vi "Read Write Exclude path.vi"(0 "path In":path, 5 "Key In":string, 7 "Exclude Path In":path[](array[path]), 11 "Error In":errorcluster, 13 "Write?":bool) -> (4 "Path Out":path, 6 "Key out":string, 8 "Exclude Path Out":path[](array[path]), 15 "Error Out":errorcluster)   [LabVIEW 2010]
uses:
  <vilib>/UTILITY/config.llb/Write Key (String).vi
  <vilib>/Utility/config.llb/Write Key (Path).vi
  <vilib>/Utility/config.llb/Read Key (String).vi
  <vilib>/Utility/config.llb/Read Key (Path).vi
  <vilib>/Utility/config.llb/NI_LVConfig.lvlib
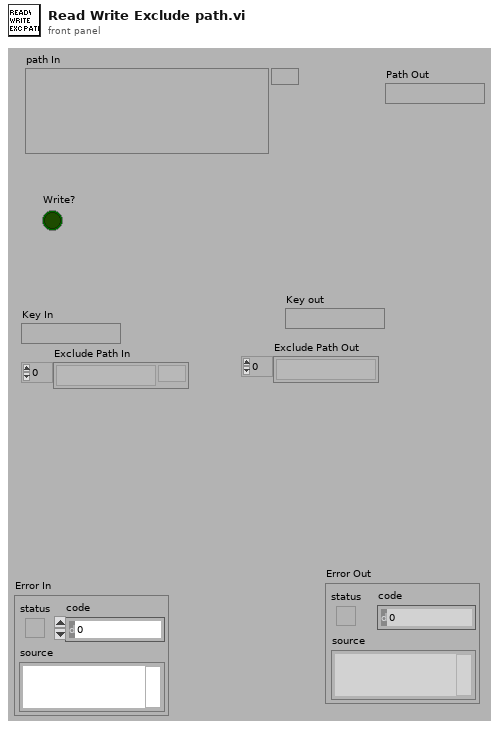
[diagram p1: front panel]
types:
  T1 = typedef "NI_LVConfig.lvlib/Config Data RefNum.ctl" = refnum<k1>
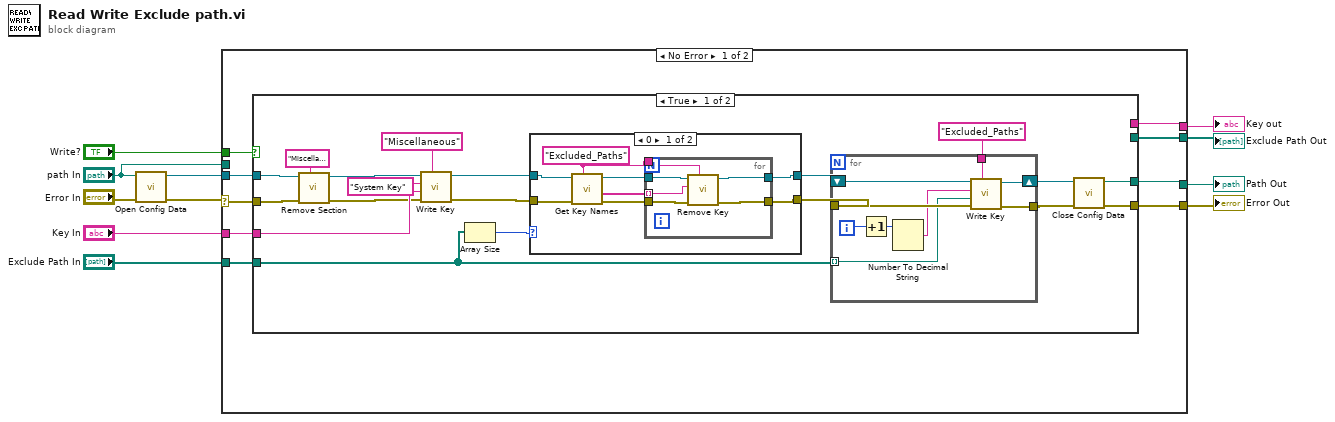
[diagram p0: block diagram]
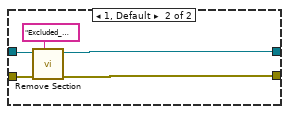
[diagram p2: hidden frame]
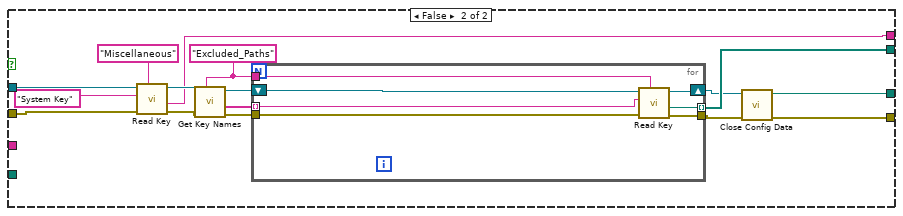
[diagram p3: hidden frame]
diagram:
  n1 = call <vilib>:"Open Config Data.vi"("error in (no error)"="Error In", "configuration file path"="path In") -> ("error out"=w10:errorcluster, "refnum"=w9:T1)  [unwired: 7 in, 1 out]
  n2 = case shown="No Error" w10 {
    selector: w10 -> [w18 _]
    tunnel: w9 -> [w19 _]
    tunnel: "Write?" -> [w20 _]
    tunnel: [w17 _] -> w7
    tunnel: "Exclude Path In" -> [w16 _]
    tunnel: "Key In" -> [w15 _]
    tunnel: [w14 _] -> w4
    tunnel: [w13 _] -> w3
    tunnel: [w12 w91] -> w1
    tunnel: "path In" -> [_ w91]
    frame No Error {
      n3 = case shown="True" w20 {
        tunnel: w19 -> [w32 w82]
        tunnel: w18 -> [w31 w83]
        tunnel: [_ w73] -> w14
        tunnel: [_ w72] -> w13
        tunnel: [w34 w69] -> w17
        tunnel: w16 -> [w26 _]
        tunnel: w15 -> [w33 _]
        tunnel: [w29 w68] -> w12
        frame True {
          n4 = call <vilib>:"Remove Section.vi"("section"="Miscellaneous", "error in (no error)"=w31, "refnum"=w32) -> ("error out"=w27:errorcluster, "refnum out"=w28:T1)  [unwired: 6 in, 1 out]
          n5 = call-poly <vilib>:"Write Key.vi"("section"="Miscellaneous", "error in (no error)"=w27, "value"=w33, "key"="System Key", "refnum"=w28) -> ("error out"=w23:errorcluster, "refnum out"=w25:T1)  [unwired: 4 in, 1 out]
          n6 = Array Size(array=w26) -> (size(s)=w21:i32)
          n7 = case shown="0" w21 {
            tunnel: w25 -> [w46 w57]
            tunnel: [w44 w56] -> w24
            tunnel: w23 -> [w47 w55]
            tunnel: [w42 w54] -> w22
            frame 0 {
              w40 = "Excluded_Paths" ("section")
              n8 = call <vilib>:"Get Key Names.vi"("section"=w40, "error in (no error)"=w47, "refnum"=w46) -> ("error out"=w43:errorcluster, "key names"=w41:string[], "refnum out"=w45:T1)  [unwired: 5 in, 1 out]
              n9 = for {
                tunnel: [w52] -> w44
                tunnel: w45 -> [w53]
                tunnel: w43 -> [w51]
                tunnel: [w50] -> w42
                tunnel: w41 -> [w49] mode=indexing
                tunnel: w40 -> [w48]
                n10 = call <vilib>:"Remove Key.vi"("section"=w48, "error in (no error)"=w51, "key"=w49, "refnum"=w53) -> ("error out"=w50:errorcluster, "refnum out"=w52:T1)  [unwired: 5 in, 1 out]
              }
            }
            frame 1, Default {
              n11 = call <vilib>:"Remove Section.vi"("section"="Excluded_Paths", "error in (no error)"=w55, "refnum"=w57) -> ("error out"=w54:errorcluster, "refnum out"=w56:T1)  [unwired: 6 in, 1 out]
            }
          }
          n12 = for {
            shift-right: [w64] -> w35
            shift-left: w24 -> [w67]
            tunnel: w22 -> [w66]
            tunnel: "Excluded_Paths" ("section") -> [w65]
            tunnel: [w63] -> w36
            tunnel: w26 -> [w62] mode=indexing
            i -> [w61]
            n13 = Increment(x=w61) -> (x+1=w60:i32)
            n14 = Number To Decimal String(number=w60) -> (decimal integer string=w59:string)  [unwired: 1 in]
            n15 = call-poly <vilib>:"Write Key.vi"("section"=w65, "error in (no error)"=w66, "value"=w62, "key"=w59, "refnum"=w67) -> ("error out"=w63:errorcluster, "refnum out"=w64:T1)  [unwired: 4 in, 1 out]
          }
          n16 = call <vilib>:"Close Config Data.vi"("error in (no error)"=w36, "refnum"=w35) -> ("error out"=w34:errorcluster, "file path"=w29:path)  [unwired: 8 in]
        }
        frame False {
          w74 = "Excluded_Paths" ("section")
          n17 = call-poly <vilib>:"Read Key.vi"("section"="Miscellaneous", "error in (no error)"=w83, "key"="System Key", "refnum"=w82) -> ("error out"=w78:errorcluster, "value"=w73:string, "refnum out"=w79:T1)  [unwired: 4 in, 1 out]
          n18 = call <vilib>:"Get Key Names.vi"("section"=w74, "error in (no error)"=w78, "refnum"=w79) -> ("error out"=w76:errorcluster, "key names"=w75:string[], "refnum out"=w77:T1)  [unwired: 5 in, 1 out]
          n19 = for {
            shift-right: [w86] -> w70
            shift-left: w77 -> [w90]
            tunnel: w76 -> [w89]
            tunnel: w75 -> [w88] mode=indexing
            tunnel: w74 -> [w87]
            tunnel: [w85] -> w71
            tunnel: [w84] -> w72 mode=indexing
            n20 = call-poly <vilib>:"Read Key.vi"("section"=w87, "error in (no error)"=w89, "key"=w88, "refnum"=w90) -> ("error out"=w85:errorcluster, "value"=w84:path, "refnum out"=w86:T1)  [unwired: 4 in, 1 out]
          }
          n21 = call <vilib>:"Close Config Data.vi"("error in (no error)"=w71, "refnum"=w70) -> ("error out"=w69:errorcluster, "file path"=w68:path)  [unwired: 8 in]
        }
      }
    }
    frame Error {
    }
  }
  "Error Out" <- w7
  "Key out" <- w4
  "Exclude Path Out" <- w3
  "Path Out" <- w1
